vi "LCC Is Control Loop Enabled.vi"(8 "error in (no error)":errorcluster caption="Fehler (Eingang, kein Fehler)", 11 "ChanHdl":i64) -> (0 "error out":errorcluster caption="Fehler (Ausgang)", 3 "Is Enabled":bool)   [LabVIEW 2021, in "labbCAN_Controller_API.lvlib"]
doc: "LCC_Func long LCC_CALL LCC_EnableControlLoop(dev_hdl ChanHdl, int Enable);"
uses:
  labbCAN_Controller_API.lvlib
  labbCAN_Controller_API.dll
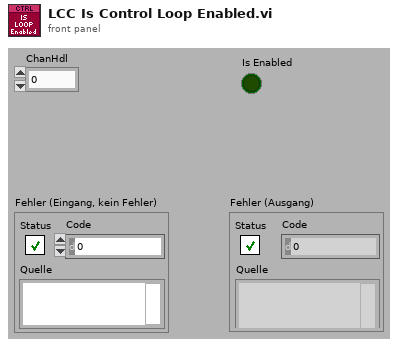
[diagram p1: front panel]
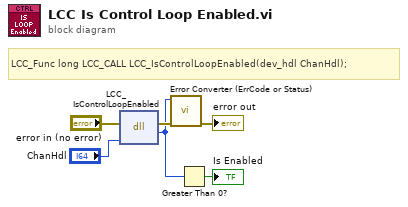
[diagram p0: block diagram]
diagram:
  # "LCC_Func long LCC_CALL LCC_IsControlLoopEnabled(dev_hdl ChanHdl);"
  n1 = dll-call lib="C:/Users/olaja/AppData/Local/CETONI_SDK/labbCAN_Controller_API.*" fn="LCC_IsControlLoopEnabled"(error in="error in (no error)", "ChanHdl"="ChanHdl") -> (error out=w4:errorcluster, "Rückgabetyp"=w1:i32)  [unwired: 3 in, 1 out]
  n2 = call "Error Converter (ErrCode or Status).vi"("error in (no error)"=w4, "error code"=w1) -> ("error out"=→"error out":errorcluster)  [unwired: 9 in]
  n3 = Greater Than 0?(x=w1) -> (x > 0?=→"Is Enabled":bool)
